vi "Thermal.vi"   [LabVIEW 2010]
doc: "An example of how you can set and get parameters from your IR-camera.\n\nNOTE: You must have IMAQ Vision, ThermoVision and GOOP installed to run this example."
uses:
  <userlib>/ThermoVision/ThermoVision.llb/Thermovision CameraTypes.ctl
  <userlib>/ThermoVision/ThermoVision.llb/ThermoVision DeviceTypes.ctl
  <userlib>/ThermoVision/ThermoVision.llb/ThermoVision CommunicationInterfaceType.ctl
  <userlib>/ThermoVision/ThermoVision Digital.llb/ThermoVision Digital ImageType.ctl
  <vilib>/Utility/file.llb/Write To Spreadsheet File (DBL).vi
types:
  T1 = typedef "ThermoVision CommunicationInterfaceType.ctl" = enum16{"File Only", "RS232", "TCP/IP(Ethernet)", "AV/C(FireWire)", "Gigabit Ethernet", "AXIS Video Server(Ethernet)"}
  T2 = typedef "ThermoVision DeviceTypes.ctl" = enum16{"No Device", "FLIR PCCard", "ITEX IC-DIG 16", "Firewire 16-bit images", "Firewire 8-bit images", "Ethernet 16-bit images", "Ethernet 8-bit images", "IR-FlashLink"}
  T3 = typedef "Thermovision CameraTypes.ctl" = enum16{"SC 2000/SC 3000", "THV320/160", "SC 1000", "ThermaCAM S40/S60", "Thermovision A20/A40", "Cumulus SC4000/SC6000", "ThermaCAM SC640", "ThermoVision A320", "ThermoVision A320G"}
  T4 = typedef "Thermovision Object Reference.ctl" = refnum<k1>
  T5 = typedef "ThermoVision Digital ImageType.ctl" = enum16{"Raw", "Absolute", "Object", "Temperature", "Raw 8 bits"}
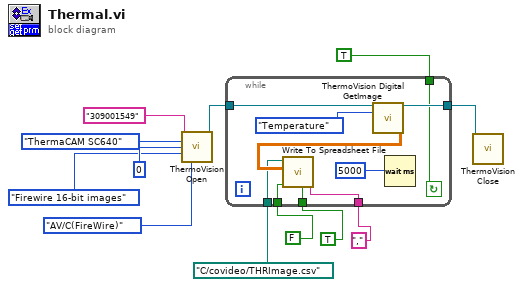
[diagram p0: block diagram]
diagram:
  n1 = call <userlib>:"ThermoVision Open.vi"("object name (unnamed)"="309001549" ("Server"), "CameraType"=Thermovision_CameraTypes."ThermaCAM SC640", "Port"=i16 0, "Device"=ThermoVision_DeviceTypes."Firewire 16-bit images", "Interface"=ThermoVision_CommunicationInterfaceType."AV/C(FireWire)") -> ("reference"=w12:T4)  [unwired: 9 in, 1 out]
  n2 = while {
    tunnel: w12 -> [w21]
    tunnel: [w20] -> w11
    tunnel: TRUE -> [w19]
    tunnel: path "C:/covideo/THRImage.csv" -> [w17]
    tunnel: FALSE -> [w16]
    tunnel: TRUE -> [w15]
    tunnel: "," -> [w14]
    stop <- w19 continue-if-true
    n3 = call <userlib>:"ThermoVision Digital GetImage.vi"("reference"=w21, "ImageType"=ThermoVision_Digital_ImageType."Temperature") -> ("duplicate reference"=w20:T4, "Image(SGL)"=w18:sgl[][])  [unwired: 8 in, 4 out]
    n4 = call-poly <vilib>:"Write To Spreadsheet File.vi"("delimiter (\\t)"=w14, "transpose? (no:F)"=w15, "append to file? (new file:F)"=w16, "2D data"=w18, "file path (dialog if empty)"=w17) -> ()  [unwired: 3 in, 1 out]
    n5 = Wait (ms)(milliseconds to wait=5000) -> ()  [unwired: 1 out]
  }
  n6 = call <userlib>:"ThermoVision Close.vi"("reference"=w11) -> ()  [unwired: 14 in, 1 out]
